vi "Retrigger.vi"(0 "VISA Resource Name":refnum<visa-resource-name>, 5 "Standard (0: IS-95A)":T1(ring), 11 "error in (no error)":errorcluster {"code" format="%.0x"}) -> (4 "VISA Resource Name Out":refnum<visa-resource-name>, 15 "error out":errorcluster {"code" format="%.0x"})   [LabVIEW 2014, in "Agilent ESG Series.lvlib"]
doc: "This VI retrigger immediate."
uses:
  Agilent ESG Series.lvlib
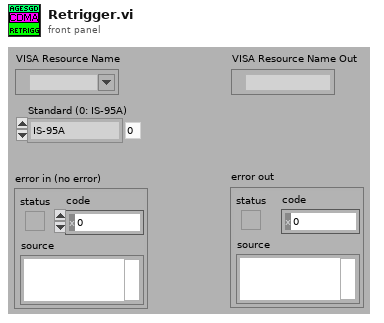
[diagram p1: front panel]
types:
  T1 = enum16{"IS-95A", "CDMA2000", "WCDMA", "Dual Arbitrary"}
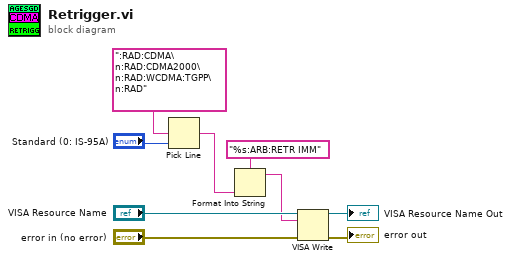
[diagram p0: block diagram]
diagram:
  n1 = Pick Line(multi-line string=":RAD:CDMA\n:RAD:CDMA2000\n:RAD:WCDMA:TGPP\n:RAD", line index="Standard (0: IS-95A)") -> (output string=w4:string)  [unwired: 1 in]
  n2 = Format Into String(format string="%s:ARB:RETR IMM", w4) -> (resulting string=w1:string)  [unwired: 2 in, 1 out]
  n3 = VISA Write(VISA resource name="VISA Resource Name", write buffer=w1, error in (no error)="error in (no error)") -> (VISA resource name out=→"VISA Resource Name Out":refnum<visa-resource-name>, error out=→"error out":errorcluster)  [unwired: 1 out]
